vi "Test Sequence.vi"() -> ()   [LabVIEW 2021]
uses:
  Source/abs_Node/Status.ctl
  Source/Test System/Test System.lvclass
  C:/Users/Tim/Documents/LabVIEW/2021/Behaviour Tree/Source/abs_System/abs_System.lvclass
  Source/Test System/Test System.lvclass/Test System.ctl
  Source/Test System/Properties/Read Log Messages.vi
  Source/abs_Node/abs_Node.lvclass
  Source/BT.lvlib
panel:
  out "Status":T1
  out "Log Messages":string[](array[string])
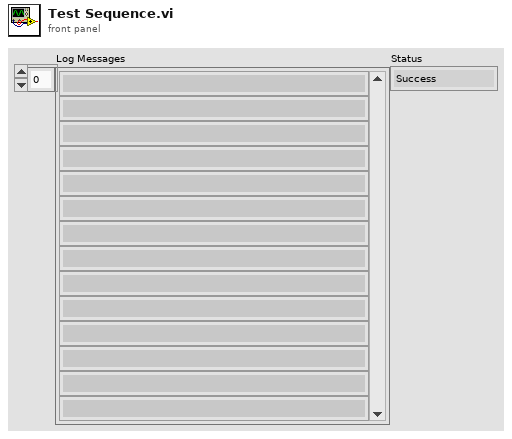
[diagram p1: front panel]
types:
  T1 = typedef "BT.lvlib/abs_Node.lvclass/Status.ctl" = enum16{"Success", "Failure", "Running"}
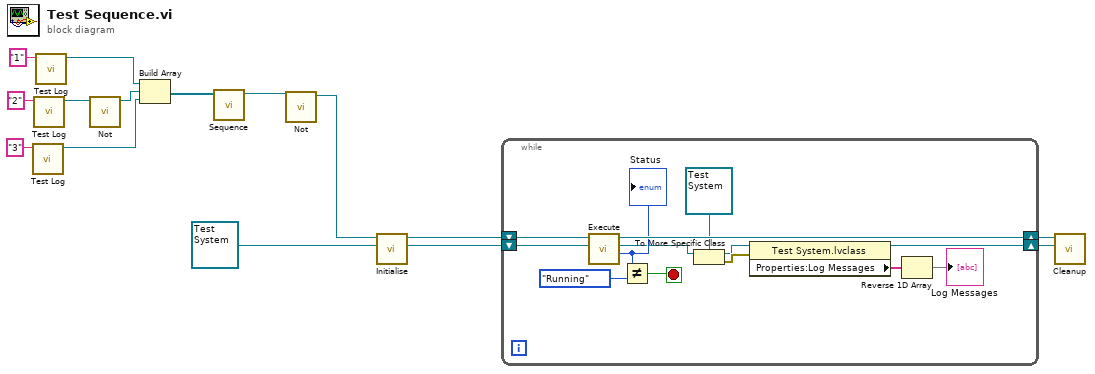
[diagram p0: block diagram]
diagram:
  n1 = call "Test Log.vi"("Message"="3") -> ("BT.lvlib:abs_Node.lvclass"=w3:refnum<class "abs_Node.lvclass">)  [unwired: 10 in]
  n2 = call "Test Log.vi"("Message"="2") -> ("BT.lvlib:abs_Node.lvclass"=w5:refnum<class "abs_Node.lvclass">)  [unwired: 10 in]
  n3 = call "Test Log.vi"("Message"="1") -> ("BT.lvlib:abs_Node.lvclass"=w9:refnum<class "abs_Node.lvclass">)  [unwired: 10 in]
  n4 = call "Not.vi"("Node In"=w5) -> ("Node"=w4:refnum<class "abs_Node.lvclass">)  [unwired: 10 in]
  n5 = Build Array(w9, w4, w3) -> (w10:refnum<class "abs_Node.lvclass">[])
  n6 = call "Sequence.vi"("Nodes"=w10) -> ("Node"=w2:refnum<class "abs_Node.lvclass">)  [unwired: 10 in]
  n7 = call "Not.vi"("Node In"=w2) -> ("Node"=w1:refnum<class "abs_Node.lvclass">)  [unwired: 10 in]
  n8 = call-dynamic "Initialise.vi"("System In"=refnum<class "Test System.lvclass"> refnum ("Test System.lvclass"), "Node in"=w1) -> ("System Out"=w13:refnum<class "abs_System.lvclass">, "Node out"=w14:refnum<class "abs_Node.lvclass">)  [unwired: 7 in, 1 out]
  n9 = while {
    shift-right: [w26] -> w12
    shift-left: w14 -> [w28]
    shift-right: [w22] -> w11
    shift-left: w13 -> [w27]
    stop <- w23 stop-if-true
    n10 = call-dynamic "Execute.vi"("System In"=w27, "Node in"=w28) -> ("Status"=w25:T1, "System Out"=w20:refnum<class "abs_System.lvclass">, "Node out"=w26:refnum<class "abs_Node.lvclass">)  [unwired: 6 in, 1 out]
    "Status" <- w25
    n11 = Not Equal?(x=w25, y=Status."Running") -> (x != y?=w23:bool)
    n12 = To More Specific Class(target class=refnum<class "Test System.lvclass"> refnum ("Test System.lvclass"), reference=w20) -> (specific class reference=w19:refnum<class "Test System.lvclass">, error out=w21:errorcluster)  [unwired: 1 in]
    n13 = property class="Test System.lvclass"(reference=w19, error in=w21) -> (reference out=w22:refnum<class "Test System.lvclass">, "Properties:Log Messages"=w17:string[])  [unwired: 1 out]
    n14 = Reverse 1D Array(array=w17) -> (reversed array=→"Log Messages":string[])
  }
  n15 = call-dynamic "Cleanup.vi"("System In"=w11, "Node in"=w12) -> ()  [unwired: 7 in, 3 out]
